vi "Create From WhileLoop Reference.vi"(8 "error in (no error)":errorcluster, 11 "Structure":refnum<vi>) -> (0 "error out":errorcluster, 3 "CSM-Helper.lvclass":refnum<class "CSM-Helper.lvclass">)   [LabVIEW 2017, in "CSM-Helper.lvclass"]
doc: "### Create From WhileLoop Reference.vi\n\n-- <b>Controls</b> --\n- <b>Structure</b>:\n\n-- <b>Indicators</b> --\n- <b>CSM-Helper.lvclass</b>:"
uses:
  CSM-Helper.lvclass
  CSM-Helper.lvclass/CSM-Helper.ctl
  Utility/CSM-Helper Utility.lvlib
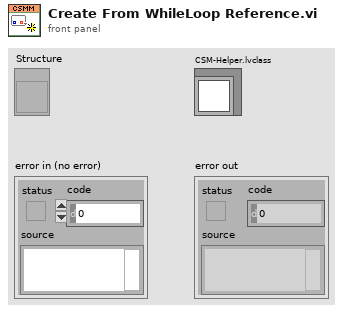
[diagram p1: front panel]
types:
  T1 = typedef "CSM-Helper Utility.lvlib/CSM Basic Refs.ctl" = cluster{"VI":refnum<vi>, "While Loop":refnum<vi>, "Case Structure":refnum<vi>, "Parse State Queue":refnum<vi>, "Event Structure":refnum<vi>, "Type":T2, "InLvlibp":bool}
  T2 = typedef "CSM-Helper Utility.lvlib/CSM Module Type.ctl" = enum16{"Not a CSM", "JKISM", "CSM"}
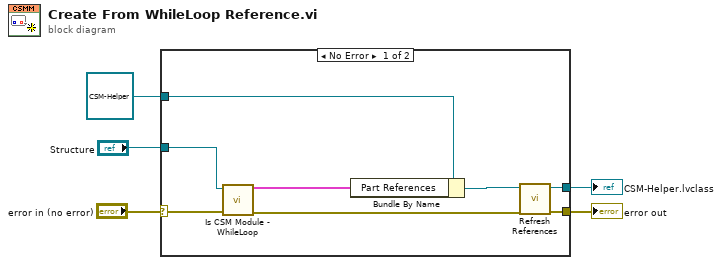
[diagram p0: block diagram]
diagram:
  n1 = case shown="No Error" "error in (no error)" {
    selector: "error in (no error)" -> [w9 w15]
    tunnel: [w10 w15] -> w5
    tunnel: [w11 w14] -> w4
    tunnel: refnum<class "CSM-Helper.lvclass"> refnum ("JKI SM") -> [w13 w14]
    tunnel: "Structure" -> [w8 _]
    frame No Error {
      n2 = call "Is CSM Module - WhileLoop.vi"("error in (no error)"=w9, "WhileLoop in"=w8) -> ("error out"=w7:errorcluster, "CSM Basic Refs"=w6:T1)  [unwired: 6 in, 2 out]
      n3 = Bundle By Name(cluster=w13, "Part References"=w6) -> (w12:refnum<class "CSM-Helper.lvclass">)
      n4 = call "Refresh References.vi"("error in (no error)"=w7, "CSM-Helper in"=w12) -> ("error out"=w10:errorcluster, "CSM-Helper out"=w11:refnum<class "CSM-Helper.lvclass">)  [unwired: 8 in]
    }
    frame Error {
    }
  }
  "error out" <- w5
  "CSM-Helper.lvclass" <- w4
